vi "add scan field(SubVI).vi"(6 "limit":T1, 10 "字符串":string) -> (0 "布尔 3":bool, 2 "连接的字符串":string)   [LabVIEW 2019, in "Add Seq.lvlib"]
uses:
  Add Seq.lvlib
  ctl/limit.ctl
  SubVI.lvlib
panel:
  in  "Number of Step":i32=2 min=0 max=70001
  in  "Step Delay(secs)":dbl
  in  "Increments(Oe)":dbl=10.0
  in  "cancel":bool
  in  "ok":bool
  in  "Approach":i32(ring)=3 items=["Linear", "NoOvershoot", "Oscillate", "Sweep"]
  in  "End Mode":i32(ring) items=["Persistent", "Driven"]
  in  "Rate(Oe/secs)":dbl=100.0 min=0.0 max=200.0
  in  "Final Field(Oe)":dbl=1000.0 min=-70000.0 max=70000.0
  in  "Initial Field(Oe)":dbl min=-70000.0 max=70000.0
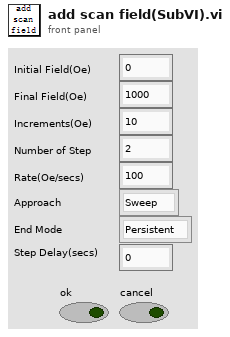
[diagram p1: front panel]
types:
  T1 = typedef "limit.ctl" = cluster{"Field limit":dbl, "Field rate limit":dbl, "Temp limit":dbl, "Temp low limit":dbl, "Temp rate limit ":dbl}
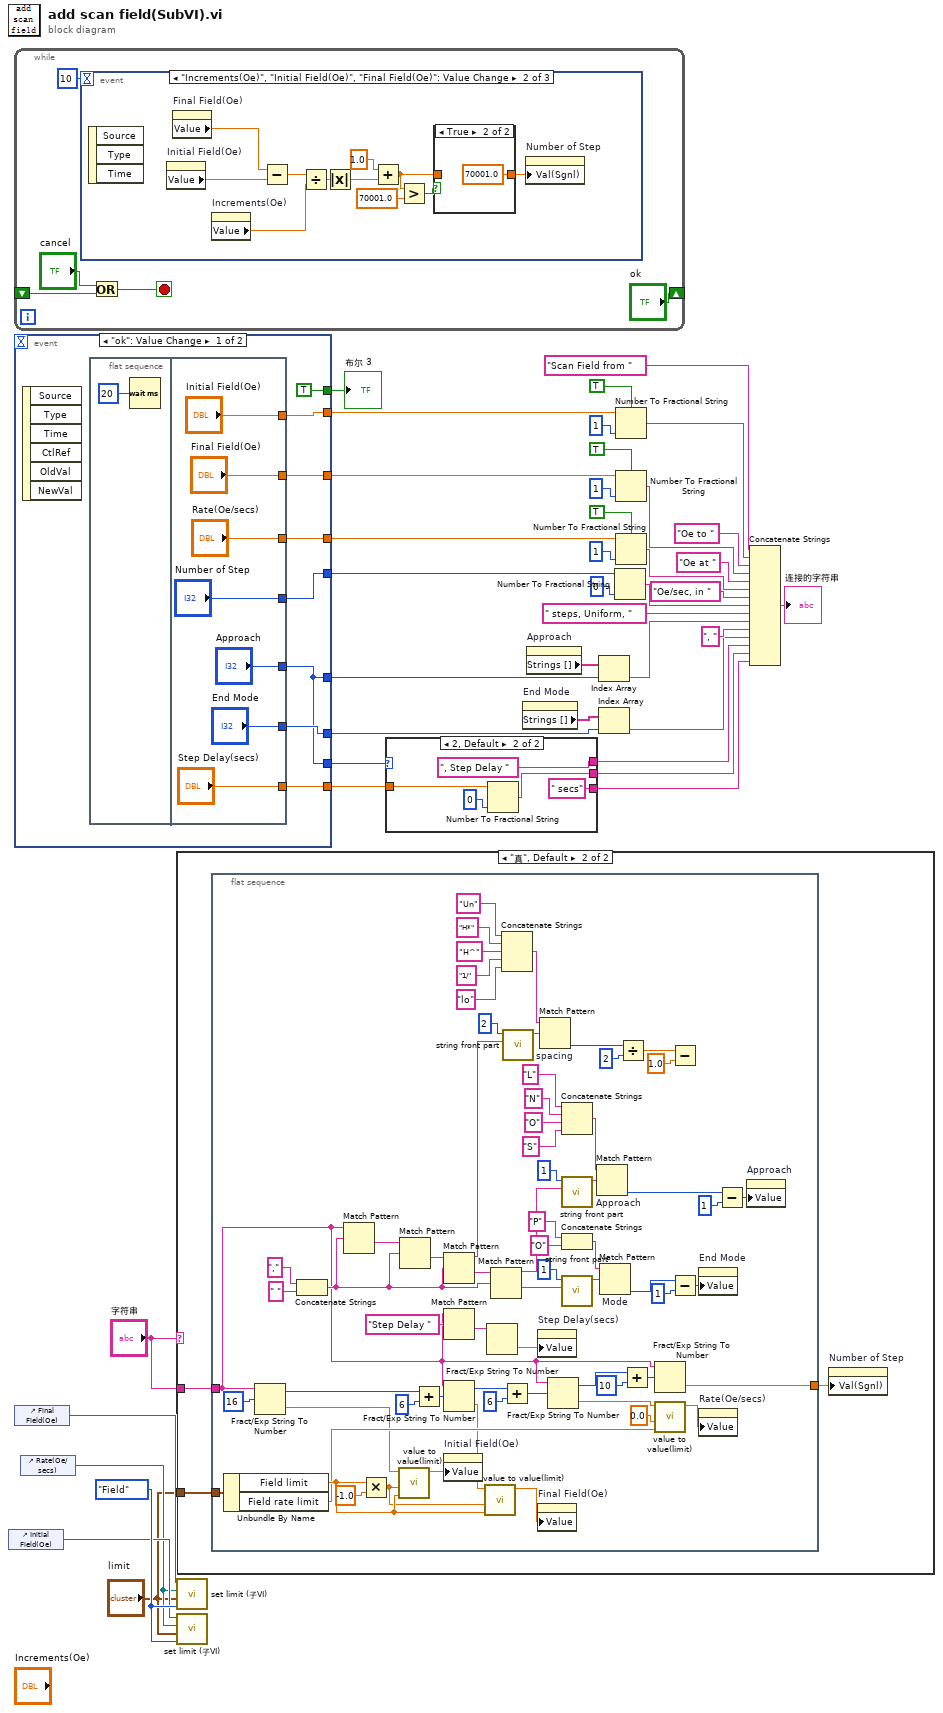
[diagram p0: block diagram]
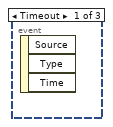
[diagram p3: hidden frame]
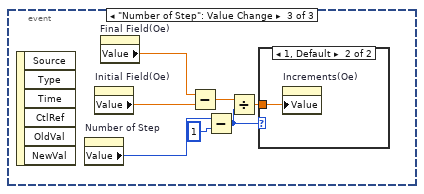
[diagram p5: hidden frame]
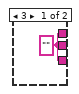
[diagram p7: hidden frame]
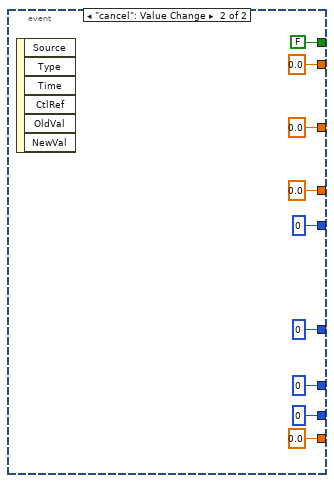
[diagram p8: hidden frame]
diagram:
  w5 = enum16{"Field", "Temp"}."Field" ("Temp or Field")
  n1 = control-ref of="Initial Field(Oe)"() -> (w4:refnum<vi>)
  n2 = while {
    shift-right: ["ok"] -> _
    shift-left: _ -> [w41]
    stop <- w43 stop-if-true
    n3 = event shown="[1] \"Increments(Oe)\", \"Initial Field(Oe)\", \"Final Field(Oe)\": Value Change" {
      selector: _ -> [_ _ _]
      dyn-events: _ -> [_ _ _]
      timeout: 10 -> [_ _ _]
      event Timeout {
        n4 = event-data() -> ()  [unwired: 1 in, 3 out]
      }
      event "Increments(Oe)", "Initial Field(Oe)", "Final Field(Oe)": Value Change {
        n5 = event-data() -> ()  [unwired: 1 in, 3 out]
        n6 = property on="Initial Field(Oe)" class="DigNum (strict)"() -> ("Value"=w55:dbl)  [unwired: 2 in, 2 out]
        n7 = property on="Final Field(Oe)" class="DigNum (strict)"() -> ("Value"=w56:dbl)  [unwired: 2 in, 2 out]
        n8 = property on="Increments(Oe)" class="DigNum (strict)"() -> ("Value"=w53:dbl)  [unwired: 2 in, 2 out]
        n9 = Subtract(x=w56, y=w55) -> (x-y=w54:dbl)
        n10 = Divide(x=w54, y=w53) -> (x/y=w51:dbl)
        n11 = Absolute Value(x=w51) -> (abs(x)=w50:dbl)
        n12 = Add(x=1.0, y=w50) -> (x+y=w47:dbl)
        n13 = Greater?(x=w47, y=70001.0) -> (0:w48:bool)
        n14 = case shown="True" w48 {
          tunnel: w47 -> [w57 _]
          tunnel: [w57 70001.0] -> w46
          frame False {
          }
          frame True {
          }
        }
        n15 = property on="Number of Step" class="DigNum (strict)"("Val(Sgnl)"=w46) -> ()  [unwired: 2 in, 2 out]
      }
      event "Number of Step": Value Change {
        n16 = event-data() -> ()  [unwired: 1 in, 6 out]
        n17 = property on="Number of Step" class="DigNum (strict)"() -> ("Value"=w62:i32)  [unwired: 2 in, 2 out]
        n18 = property on="Initial Field(Oe)" class="DigNum (strict)"() -> ("Value"=w64:dbl)  [unwired: 2 in, 2 out]
        n19 = property on="Final Field(Oe)" class="DigNum (strict)"() -> ("Value"=w65:dbl)  [unwired: 2 in, 2 out]
        n20 = Subtract(x=w65, y=w64) -> (x-y=w63:dbl)
        n21 = Subtract(x=w62, y=1) -> (x-y=w59:i32)
        n22 = Divide(x=w63, y=w59) -> (x/y=w60:dbl)
        n23 = case shown="1, Default" w59 {
          tunnel: w60 -> [_ w66]
          frame 0 {
          }
          frame 1, Default {
            n24 = property on="Increments(Oe)" class="DigNum (strict)"("Value"=w66) -> ()  [unwired: 2 in, 2 out]
          }
        }
      }
    }
    n25 = Or(x="cancel", y=w41) -> (x .or. y?=w43:bool)
  }
  n26 = event shown="[0] \"ok\": Value Change" {
    selector: _ -> [_ _]
    dyn-events: _ -> [_ _]
    timeout: _ -> [_ _]
    tunnel: [w74 0.0 ("Field 2")] -> w29
    tunnel: [w73 0.0 ("Rate输入")] -> w26
    tunnel: [w72 0.0 ("Field")] -> w38
    tunnel: [TRUE FALSE] -> w40
    tunnel: [w67 0 ("Number of Step")] -> w23
    tunnel: [w70 0 ("Mode输入")] -> w19
    tunnel: [w68 0 ("Approach输入")] -> w16
    tunnel: [w69 0.0 ("Step Delay(secs)")] -> w10
    tunnel: [w68 0 ("Approach")] -> w8
    event "ok": Value Change {
      n27 = event-data() -> ()  [unwired: 1 in, 6 out]
      n28 = flat-sequence {
        tunnel: ["Final Field(Oe)"] -> w74
        tunnel: ["Rate(Oe/secs)"] -> w73
        tunnel: ["Initial Field(Oe)"] -> w72
        tunnel: ["End Mode"] -> w70
        tunnel: ["Step Delay(secs)"] -> w69
        tunnel: ["Approach"] -> w68
        tunnel: ["Number of Step"] -> w67
        frame #0 {
          n29 = Wait (ms)(milliseconds to wait=u32 20 ("等待时间（毫秒）")) -> ()  [unwired: 1 out]
        }
        frame #1 {
        }
      }
    }
    event "cancel": Value Change {
      n30 = event-data() -> ()  [unwired: 1 in, 6 out]
    }
  }
  "布尔 3" <- w40
  n31 = control-ref of="Final Field(Oe)"() -> (w3:refnum<vi>)
  n32 = control-ref of="Rate(Oe/secs)"() -> (w2:refnum<vi>)
  n33 = case shown="\"真\", Default" "字符串" {
    tunnel: "字符串" -> [_ w93]
    tunnel: "limit" -> [_ w92]
    frame "" {
    }
    frame "真", Default {
      n34 = flat-sequence {
        tunnel: [w111] -> w94
        tunnel: w93 -> [w107]
        tunnel: w92 -> [w106]
        frame #0 {
          n35 = Unbundle By Name(w106) -> ("Field limit"=w104:dbl, "Field rate limit"=w102:dbl)
          n36 = Fract/Exp String To Number(string=w107, offset=16 ("偏移量")) -> (offset past number=w158:i32, number=w96:dbl)  [unwired: 2 in]
          n37 = Concatenate Strings("," ("字符串"), " " ("字符串")) -> (w119:string)
          n38 = Match Pattern(string=w107, regular expression=w119) -> (after substring=w160:string)  [unwired: 1 in, 3 out]
          n39 = Multiply(x=w104, y=-1.0) -> (x*y=w103:dbl)
          n40 = call "value to value(limit).vi"("high limit"=w104, "low limit"=w103, "数值 in"=w96) -> ("数值 out"=w95:dbl)  [unwired: 8 in]
          n41 = Match Pattern(string=w160, regular expression=w119) -> (after substring=w135:string)  [unwired: 1 in, 3 out]
          n42 = Add(x=w158, y=6) -> (x+y=w157:i32)
          n43 = Match Pattern(string=w135, regular expression=w119) -> (before substring=w134:string, after substring=w120:string)  [unwired: 1 in, 2 out]
          n44 = Match Pattern(string=w107, regular expression="Step Delay ") -> (after substring=w115:string)  [unwired: 1 in, 3 out]
          n45 = Fract/Exp String To Number(string=w107, offset=w157) -> (offset past number=w140:i32, number=w98:dbl)  [unwired: 2 in]
          n46 = property on="Initial Field(Oe)" class="DigNum (strict)"("Value"=w95) -> ()  [unwired: 2 in, 2 out]
          n47 = call "value to value(limit).vi"("high limit"=w104, "low limit"=w103, "数值 in"=w98) -> ("数值 out"=w97:dbl)  [unwired: 8 in]
          n48 = Fract/Exp String To Number(string=w115) -> (number=w113:dbl)  [unwired: 3 in, 1 out]
          n49 = Match Pattern(string=w120, regular expression=w119) -> (before substring=w118:string, after substring=w117:string)  [unwired: 1 in, 2 out]
          n50 = Concatenate Strings("Un" ("字符串"), "H*" ("字符串"), "H^" ("字符串"), "1/" ("字符串"), "lo" ("字符串")) -> (w126:string)
          n51 = Add(x=w140, y=6) -> (x+y=w138:i32)
          n52 = call "string front part.vi"("字符串"=w134, "偏移量(0)"=2) -> ("result string"=w132:string)  [unwired: 9 in]
          n53 = property on="Step Delay(secs)" class="DigNum (strict)"("Value"=w113) -> ()  [unwired: 2 in, 2 out]
          n54 = property on="Final Field(Oe)" class="DigNum (strict)"("Value"=w97) -> ()  [unwired: 2 in, 2 out]
          n55 = Match Pattern "spacing"(string=w126, regular expression=w132) -> (offset past match=w125:i32)  [unwired: 1 in, 3 out]
          n56 = Fract/Exp String To Number(string=w107, offset=w138) -> (offset past number=w121:i32, number=w100:dbl)  [unwired: 2 in]
          n57 = Concatenate Strings("L" ("字符串"), "N" ("字符串"), "O" ("字符串"), "S" ("字符串")) -> (w150:string)
          n58 = call "string front part.vi"("字符串"=w118, "偏移量(0)"=1) -> ("result string"=w154:string)  [unwired: 9 in]
          n59 = Concatenate Strings("P" ("字符串"), "O" ("字符串")) -> (w145:string)
          n60 = call "string front part.vi"("字符串"=w117, "偏移量(0)"=1) -> ("result string"=w148:string)  [unwired: 9 in]
          n61 = Match Pattern "Approach"(string=w150, regular expression=w154) -> (offset past match=w109:i32)  [unwired: 1 in, 3 out]
          n62 = Match Pattern "Mode"(string=w145, regular expression=w148) -> (offset past match=w144:i32)  [unwired: 1 in, 3 out]
          n63 = Divide(x=w125, y=2) -> (x/y=w123:dbl)
          n64 = Add(x=w121, y=10) -> (x+y=w136:i32)
          n65 = Fract/Exp String To Number(string=w107, offset=w136) -> (number=w111:dbl)  [unwired: 2 in, 1 out]
          n66 = call "value to value(limit).vi"("high limit"=w102, "low limit"=0.0, "数值 in"=w100) -> ("数值 out"=w99:dbl)  [unwired: 8 in]
          n67 = Subtract(x=w123, y=1.0) -> ()  [unwired: 1 out]
          n68 = Subtract(x=w144, y=1) -> (x-y=w112:i32)
          n69 = property on="End Mode" class="Ring (strict)"("Value"=w112) -> ()  [unwired: 2 in, 2 out]
          n70 = property on="Rate(Oe/secs)" class="DigNum (strict)"("Value"=w99) -> ()  [unwired: 2 in, 2 out]
          n71 = Subtract(x=w109, y=1) -> (x-y=w108:i32)
          n72 = property on="Approach" class="Ring (strict)"("Value"=w108) -> ()  [unwired: 2 in, 2 out]
        }
      }
      n73 = property on="Number of Step" class="DigNum (strict)"("Val(Sgnl)"=w94) -> ()  [unwired: 2 in, 2 out]
    }
  }
  n74 = call "set limit (子VI).vi"("Temp or Field"=w5, "limit"="limit", "rate"=w2, "value"=w3) -> ()  [unwired: 8 in]
  n75 = call "set limit (子VI).vi"("Temp or Field"=w5, "limit"="limit", "rate"=w2, "value"=w4) -> ()  [unwired: 8 in]
  n76 = case shown="2, Default" w8 {
    tunnel: [w161 ", Step Delay " ("字符串")] -> w12
    tunnel: [w161 " secs" ("字符串")] -> w11
    tunnel: w10 -> [_ w164]
    tunnel: [w161 w163] -> w9
    frame 3 {
      w161 = ""
    }
    frame 2, Default {
      n77 = Number To Fractional String(number=w164, precision (6)=i16 0 ("精度(6)")) -> (F-format string=w163:string)  [unwired: 2 in]
    }
  }
  n78 = property on="End Mode" class="Ring (strict)"() -> ("Strings []"=w20:string[])  [unwired: 2 in, 2 out]
  n79 = property on="Approach" class="Ring (strict)"() -> ("Strings []"=w17:string[])  [unwired: 2 in, 2 out]
  n80 = Index Array(array=w17, index=w16) -> (element=w13:string)
  n81 = Index Array(array=w20, index=w19) -> (element=w14:string)
  n82 = Number To Fractional String(number=w23, precision (6)=i16 0 ("精度(6)")) -> (F-format string=w22:string)  [unwired: 2 in]
  n83 = Number To Fractional String(use system decimal point (T)=TRUE ("使用系统小数点(T)"), number=w38, precision (6)=i16 1 ("精度(6)")) -> (F-format string=w36:string)  [unwired: 1 in]
  n84 = Number To Fractional String(use system decimal point (T)=TRUE ("使用系统小数点(T)"), number=w29, precision (6)=i16 1 ("精度(6)")) -> (F-format string=w31:string)  [unwired: 1 in]
  n85 = Number To Fractional String(use system decimal point (T)=TRUE ("使用系统小数点(T)"), number=w26, precision (6)=i16 1 ("精度(6)")) -> (F-format string=w25:string)  [unwired: 1 in]
  n86 = Concatenate Strings("Scan Field from " ("字符串"), w36, "Oe to " ("字符串"), w31, "Oe at " ("字符串"), w25, "Oe/sec, in " ("字符串"), w22, " steps, Uniform, " ("字符串"), w13, ", " ("字符串"), w14, w12, w9, w11) -> (→"连接的字符串":string)
